vi "Throw Unknown Setting Error.vi"(7 "source vi name":string, 8 "error in (no error)":errorcluster, 9 "value":string, 10 "key":string) -> (0 "error out":errorcluster)   [LabVIEW 2023, in "UDPlog.lvlib" / "UDPlog Transceiver.lvclass"]
uses:
  UDPlog Transceiver.lvclass
  UDPlog Transceiver.lvclass/UDPlog Transceiver.ctl
  <vilib>/NI/Memory Manager/Static Errors.lvlib
  Typedefs/Errors.ctl
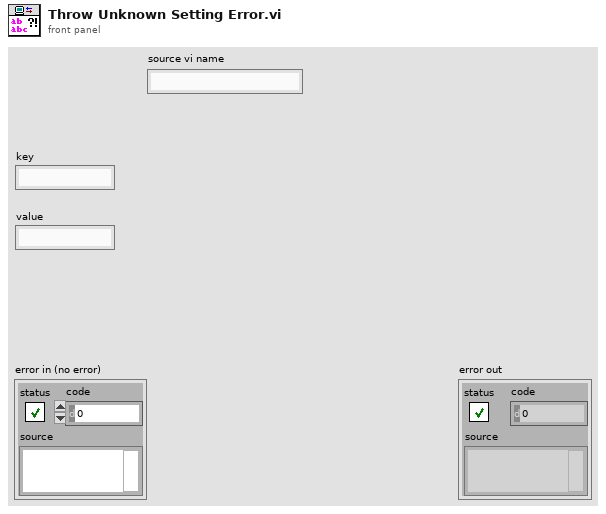
[diagram p1: front panel]
types:
  T1 = typedef "UDPlog.lvlib/UDPlog Transceiver.lvclass/Errors.ctl" = enum16{"Unknown Datagram", "Size Mismatch", "Unknown Setting"}
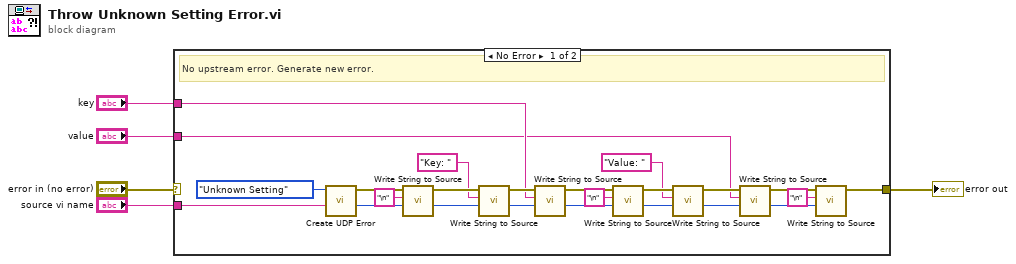
[diagram p0: block diagram]
diagram:
  n1 = case shown="No Error" "error in (no error)" {
    selector: "error in (no error)" -> [_ w30]
    tunnel: [w7 w30] -> w2
    tunnel: "value" -> [w11 _]
    tunnel: "key" -> [w20 _]
    tunnel: "source vi name" -> [w29 _]
    frame No Error {
      # "No upstream error. Generate new error."
      n2 = call "Create UDP Error.vi"("source vi name"=w29, "error"=Errors."Unknown Setting" ("Error")) -> ("offset"=w6:i32, "error out"=w26:errorcluster)  [unwired: 8 in]
      n3 = call <vilib>:"Write String to Source.vi"("offset"=w6, "string"="\n", "error in"=w26) -> ("new offset"=w24:i32, "error out"=w25:errorcluster)  [unwired: 7 in]
      n4 = call <vilib>:"Write String to Source.vi"("offset"=w24, "string"="Key: ", "error in"=w25) -> ("new offset"=w21:i32, "error out"=w22:errorcluster)  [unwired: 7 in]
      n5 = call <vilib>:"Write String to Source.vi"("offset"=w21, "string"=w20, "error in"=w22) -> ("new offset"=w17:i32, "error out"=w18:errorcluster)  [unwired: 7 in]
      n6 = call <vilib>:"Write String to Source.vi"("offset"=w17, "string"="\n", "error in"=w18) -> ("new offset"=w15:i32, "error out"=w16:errorcluster)  [unwired: 7 in]
      n7 = call <vilib>:"Write String to Source.vi"("offset"=w15, "string"="Value: ", "error in"=w16) -> ("new offset"=w13:i32, "error out"=w12:errorcluster)  [unwired: 7 in]
      n8 = call <vilib>:"Write String to Source.vi"("offset"=w13, "string"=w11, "error in"=w12) -> ("new offset"=w8:i32, "error out"=w9:errorcluster)  [unwired: 7 in]
      n9 = call <vilib>:"Write String to Source.vi"("offset"=w8, "string"="\n", "error in"=w9) -> ("error out"=w7:errorcluster)  [unwired: 7 in, 1 out]
    }
    frame Error {
      # "Upstream error. Pass through."
    }
  }
  "error out" <- w2
